vi "Get RX Message.vi"(8 "error in (no error)":errorcluster, 11 "RxTx in":refnum<class "CCS_RxTx.lvclass">) -> (0 "error out":errorcluster, 2 "new msg":bool, 3 "RxTx out":refnum<class "CCS_RxTx.lvclass">)   [LabVIEW 2018, in "CCS_RxTx.lvclass"]
doc: "Pop the lastest Rx message found in the qeue"
uses:
  CCS_RxTx.lvclass
  CCS_RxTx.lvclass/CCS_RxTx.ctl
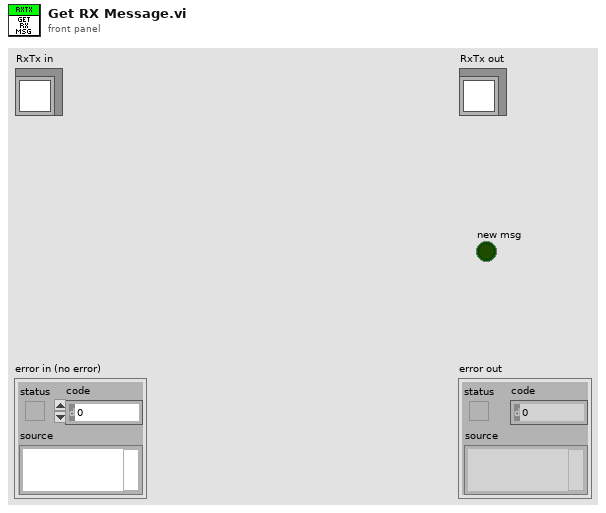
[diagram p1: front panel]
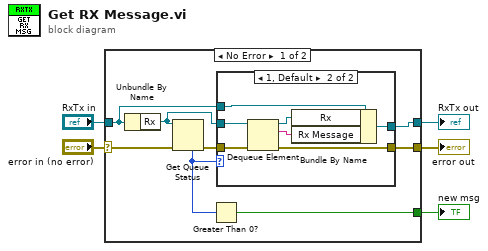
[diagram p0: block diagram]
diagram:
  n1 = case shown="No Error" "error in (no error)" {
    selector: "error in (no error)" -> [w10 w24]
    tunnel: [w8 w24] -> w2
    tunnel: [w12 w23] -> w3
    tunnel: "RxTx in" -> [w13 w23]
    tunnel: [w6 _] -> w1
    frame No Error {
      n2 = Unbundle By Name(w13) -> ("Rx"=w11:refnum<queue>)
      n3 = Get Queue Status(queue=w11, error in (no error)=w10) -> (error out=w9:errorcluster, # elements in queue=w7:i32)  [unwired: 1 in, 6 out]
      n4 = Greater Than 0?(x=w7) -> (x > 0?=w6:bool)
      n5 = case shown="1, Default" w7 {
        tunnel: w11 -> [_ w22]
        tunnel: w13 -> [w14 w21]
        tunnel: [w14 w20] -> w12
        tunnel: w9 -> [w15 w18]
        tunnel: [w15 w17] -> w8
        frame 0 {
        }
        frame 1, Default {
          n6 = Dequeue Element(queue=w22, error in (no error)=w18) -> (queue out=w16:refnum<queue>, element=w19:string, error out=w17:errorcluster)  [unwired: 1 in, 1 out]
          n7 = Bundle By Name(cluster=w21, "Rx"=w16, "Rx Message"=w19) -> (w20:refnum<class "CCS_RxTx.lvclass">)
        }
      }
    }
    frame Error {
    }
  }
  "error out" <- w2
  "RxTx out" <- w3
  "new msg" <- w1
